vi "Send Block and HT Position (SubVI).vi"(8 "HT LOC":u64[](array[numeric]), 10 "BBOX Array":u64[](array[numeric]), 11 "FPGA REF":T1) -> ()   [LabVIEW 2020]
uses:
  Controls (HOST)/FPGA REF (MWT).ctl
  <vilib>/Utility/error.llb/Error Cluster From Error Code.vi
  <vilib>/rvi/errors/niLvFpgaAdjustHostInterfaceError.vi
  <vilib>/rvi/interface/nirviMethod/nirviMethod.xnode
  <vilib>/FPGAPlugInAG/Dynamic/niLvFpga_WriteFifo_Dynamic.vi
  <vilib>/rvi/errors/niLvFpgaMergeErrorWithErrorCode.vi
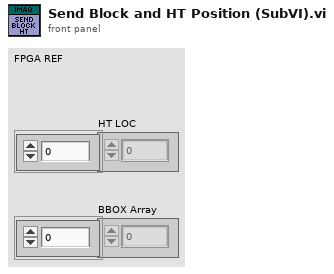
[diagram p1: front panel]
types:
  T1 = typedef "FPGA REF (MWT).ctl" = refnum<k20>
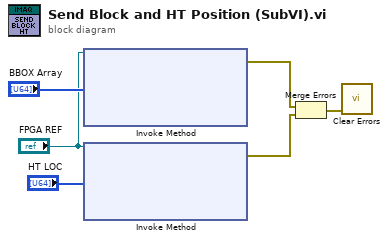
[diagram p0: block diagram]
diagram:
  n1 = xnode "Invoke Method"("FPGA VI Reference In"="FPGA REF", "Data"="BBOX Array") -> ("error out"=w2:errorcluster)  [unwired: 2 in, 2 out]
  n2 = xnode "Invoke Method"("FPGA VI Reference In"="FPGA REF", "Data"="HT LOC") -> ("error out"=w1:errorcluster)  [unwired: 2 in, 2 out]
  n3 = Merge Errors(w2, w1) -> (w3:errorcluster)
  n4 = call <vilib>:"Clear Errors.vi"("error in (no error)"=w3) -> ()  [unwired: 5 in, 2 out]
